vi "SeqnSet.vi"(1 "Sequence":refnum<class "Cohort.lvclass">[](array[class]), 3 "error in (no error)":errorcluster) -> (7 "Sequence out":refnum<class "Sequence.lvclass">, 10 "error out":errorcluster)   [LabVIEW 2012, in "Sequence.lvclass"]
uses:
  Sequence.lvclass
  Cohort.lvclass
  Sequence.lvclass/Sequence.ctl
panel:
  in  "Sequence in":refnum<class "Sequence.lvclass">
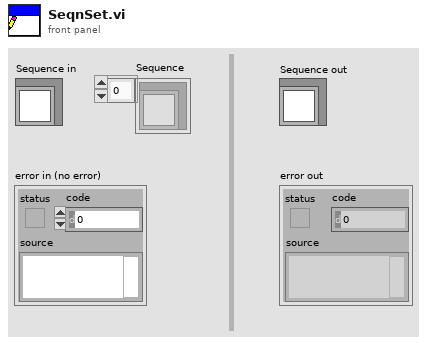
[diagram p1: front panel]
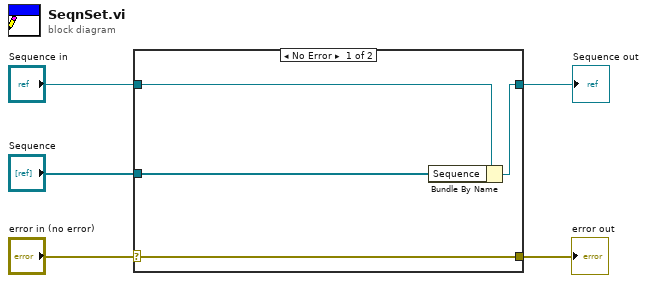
[diagram p0: block diagram]
diagram:
  n1 = case shown="No Error" "error in (no error)" {
    selector: "error in (no error)" -> [w9 w10]
    tunnel: [w9 w10] -> w4
    tunnel: [w7 w11] -> w1
    tunnel: "Sequence in" -> [w8 w11]
    tunnel: "Sequence" -> [w6 _]
    frame No Error {
      n2 = Bundle By Name(cluster=w8, "Sequence"=w6) -> (w7:refnum<class "Sequence.lvclass">)
    }
    frame Error {
    }
  }
  "error out" <- w4
  "Sequence out" <- w1
